vi "Flush Target Messages.vi"(6 "Paras In":variant, 8 "error in (no error)":errorcluster, 10 "Mail Strategy In":refnum<class "Mail Strategy.lvclass">, 11 "Simple Map Queue Group Messenger in":refnum<class "Simple Map Queue Group Messenger.lvclass">) -> (0 "error out":errorcluster, 2 "Flushed Messages":refnum<class "Message.lvclass">[](array[class]), 3 "Simple Map Queue Group Messenger out":refnum<class "Simple Map Queue Group Messenger.lvclass">)   [LabVIEW 2024, in "Simple Map Queue Group Messenger.lvclass"]
uses:
  Simple Map Queue Group Messenger.lvclass
  Ancestor Class/Messenger/Mail Strategy/Mail Strategy.lvclass
  Ancestor Class/Message/Message.lvclass
  Simple Map Queue Group Messenger.lvclass/Simple Map Queue Group Messenger.ctl
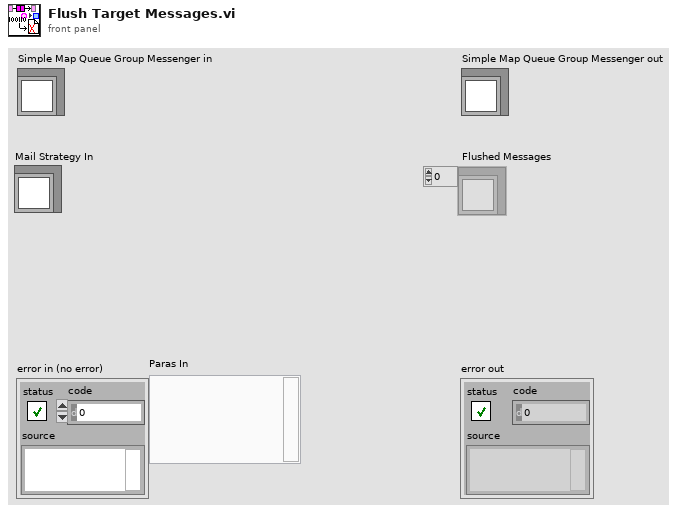
[diagram p1: front panel]
types:
  T1 = typedef "Queue Group Map.ctl" = map{i64, T2[]}
  T2 = typedef "Message Queue.ctl" = refnum<queue>
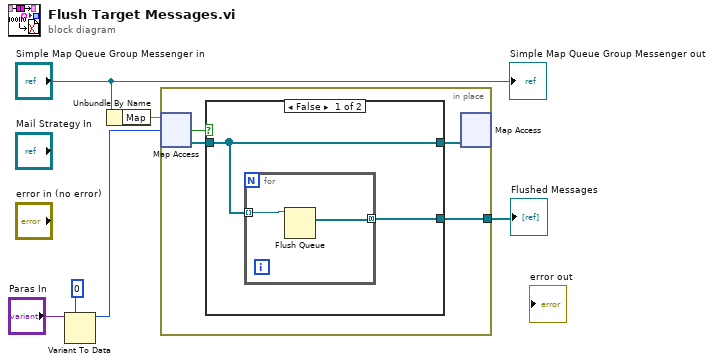
[diagram p0: block diagram]
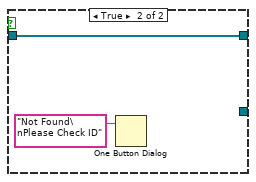
[diagram p2: hidden frame]
diagram:
  n1 = Variant To Data(type=i64 0, Variant="Paras In") -> (data=w4:i64)  [unwired: 1 in, 1 out]
  n2 = Unbundle By Name("Simple Map Queue Group Messenger in") -> ("Map"=w6:T1)
  n3 = in-place {
    in-place-border: [w7] -> w1
    n4 = in-place-map #1(w6, w4) -> (w9:T2[], w10:bool)  [unwired: 1 in]
    n5 = case shown="False" w10 {
      tunnel: w9 -> [w12 w15]
      tunnel: [w12 w15] -> w8
      tunnel: [w11 _] -> w7
      frame False {
        n6 = for {
          tunnel: w12 -> [w14] mode=indexing
          tunnel: [w13] -> w11 mode=concatenating
          n7 = Flush Queue(queue=w14) -> (remaining elements=w13:refnum<class "Message.lvclass">[])  [unwired: 1 in, 2 out]
        }
      }
      frame True {
        n8 = One Button Dialog(message="Not Found\nPlease Check ID") -> ()  [unwired: 1 in, 1 out]
      }
    }
    n9 = in-place-map #1(w8) -> ()  [unwired: 1 in, 3 out]
  }
  "Flushed Messages" <- w1
  "Simple Map Queue Group Messenger out" <- "Simple Map Queue Group Messenger in"
